vi "datatype.vi"() -> ()   [LabVIEW 2020]
panel:
  in  "Array 7":void[](array[numeric])
  out "Array 6":string[](array[string])
  in  "Array 5":string[](array[string])
  in  "Array 4":bool[](array[boolean])
  out "Array 3":bool[](array[boolean])
  out "Array 2":dbl[](array[numeric])
  in  "Array":dbl[](array[numeric])
  out "String 2":string
  in  "String":string
  out "Boolean 2":bool
  in  "Boolean":bool
  out "Numeric 2":dbl
  in  "Numeric":dbl
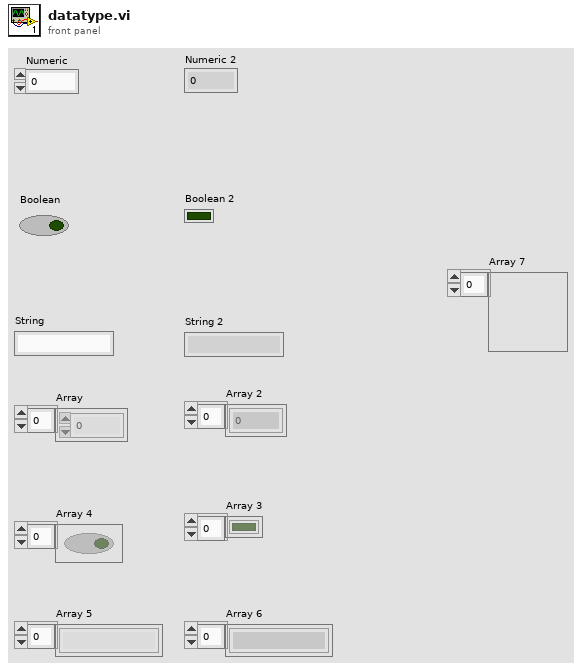
[diagram p1: front panel]
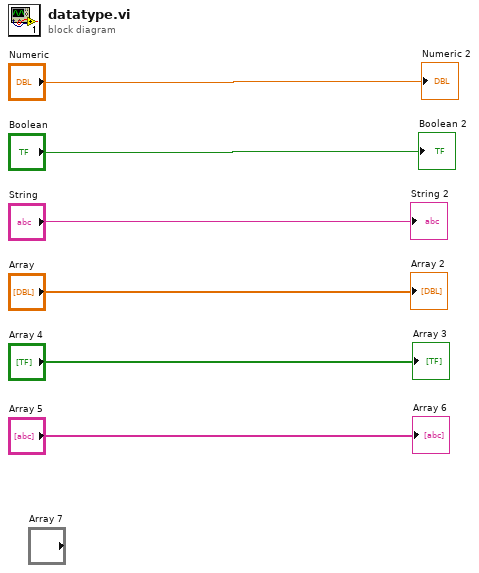
[diagram p0: block diagram]
diagram:
  "Numeric 2" <- "Numeric"
  "Boolean 2" <- "Boolean"
  "String 2" <- "String"
  "Array 2" <- "Array"
  "Array 3" <- "Array 4"
  "Array 6" <- "Array 5"
